vi "ScpiSendReplywHandle.vi"(7 "error in (no error)":errorcluster, 8 "Command":string, 10 "connection ID In":refnum<k5>) -> (0 "Error out":errorcluster, 2 "Reply":string, 3 "connection ID Out":refnum<k5>)   [LabVIEW 2009]
doc: "Sends a SCPI command to an instrument.\nWaits for the reply.\nReply string must end in NewLine character."
panel:
  in  "TCP TO":i32=1000
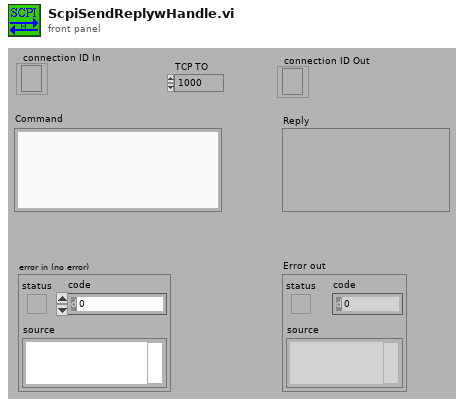
[diagram p1: front panel]
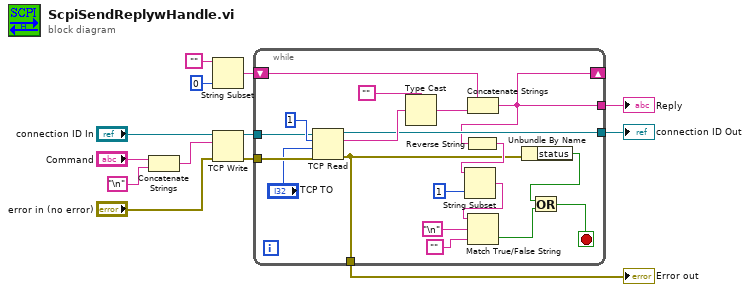
[diagram p0: block diagram]
diagram:
  n1 = Concatenate Strings("Command", "\n") -> (w12:string)
  n2 = String Subset(string="", length (rest)=0) -> (substring=w5:string)  [unwired: 1 in]
  n3 = TCP Write(connection ID="connection ID In", data in=w12, error in (no error)="error in (no error)") -> (connection ID out=w11:refnum<k5>, error out=w10:errorcluster)  [unwired: 1 in, 1 out]
  n4 = while {
    tunnel: w11 -> [w31]
    tunnel: w10 -> [w30]
    shift-right: [w19] -> _
    shift-left: w5 -> [w26]
    tunnel: [w16] -> w2
    tunnel: [w25] -> w9
    tunnel: [w19] -> w8
    stop <- w14 stop-if-true
    n5 = TCP Read(connection ID=w31, bytes to read=1, error in (no error)=w30, 9:"TCP TO") -> (connection ID out=w25:refnum<k5>, data out=w29:string, error out=w16:errorcluster)  [unwired: 1 in]
    n6 = Type Cast(type="", x=w29) -> (*(type *) &x=w27:string)
    n7 = Concatenate Strings(w26, w27) -> (w19:string)
    n8 = Reverse String(1:w19) -> (0:w24:string)
    n9 = String Subset(string=w24, length (rest)=1) -> (substring=w22:string)  [unwired: 1 in]
    n10 = Match True/False String(2:"", 3:"\n", 4:w22) -> (0:w17:bool)  [unwired: 1 out]
    n11 = Unbundle By Name(w16) -> ("status"=w15:bool)
    n12 = Or(x=w15, y=w17) -> (x .or. y?=w14:bool)
  }
  "Error out" <- w2
  "Reply" <- w8
  "connection ID Out" <- w9
